vi "Get HW Interface Inputs.vi"(8 "error in (no error)":errorcluster, 11 "Grips Robot in":refnum<class "Grips Robot.lvclass">) -> (0 "error out":errorcluster, 1 "Digital Outputs":T1, 2 "Analog Outputs":T2, 3 "Grips Robot out":refnum<class "Grips Robot.lvclass">)   [LabVIEW 2013, in "Grips Robot.lvclass"]
uses:
  Grips Robot.lvclass
  Hardware Interface/DblArrayWithName.ctl
  Hardware Interface/BoolArrayWithName.ctl
  Grips Robot.lvclass/Grips Robot.ctl
  Hardware Interface/Hardware Interface.lvclass/Hardware Interface.ctl
  Hardware Interface/Hardware Interface.lvclass
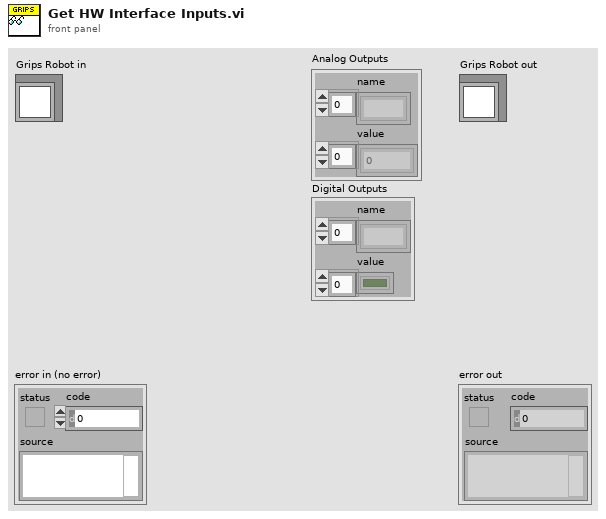
[diagram p1: front panel]
types:
  T1 = typedef "BoolArrayWithName.ctl" = cluster{"name":string[], "value":bool[]}
  T2 = typedef "DblArrayWithName.ctl" = cluster{"name":string[], "value":dbl[]}
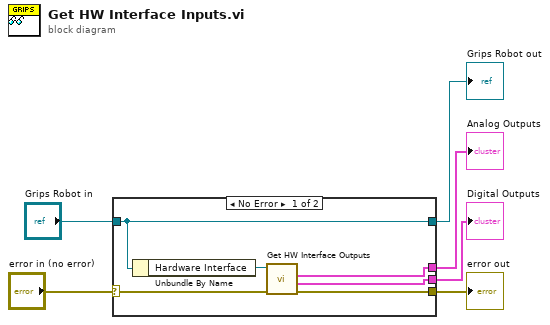
[diagram p0: block diagram]
diagram:
  n1 = case shown="No Error" "error in (no error)" {
    selector: "error in (no error)" -> [w10 w13]
    tunnel: [w9 w13] -> w5
    tunnel: [w12 w14] -> w3
    tunnel: "Grips Robot in" -> [w12 w14]
    tunnel: [w8 _] -> w2
    tunnel: [w7 _] -> w1
    frame No Error {
      n2 = Unbundle By Name(w12) -> ("Hardware Interface"=w11:refnum<class "Hardware Interface.lvclass">)
      n3 = call "Get HW Interface Outputs.vi"("error in (no error)"=w10, "Hardware Interface in"=w11) -> ("error out"=w9:errorcluster, "Digital Outputs"=w7:T1, "Analog Outputs"=w8:T2)  [unwired: 6 in, 1 out]
    }
    frame Error {
    }
  }
  "error out" <- w5
  "Grips Robot out" <- w3
  "Analog Outputs" <- w2
  "Digital Outputs" <- w1
